vi "Connect.vi"(8 "error in":errorcluster, 11 "Luminos in":refnum<class "Luminos.lvclass">) -> (0 "error out":errorcluster, 3 "Luminos out":refnum<class "Luminos.lvclass">)   [LabVIEW 2018, in "Luminos.lvlib" / "Luminos.lvclass"]
uses:
  Luminos.lvclass
  PPLs/Axis/Axis.lvlibp/Axis.lvclass
  <instrlib>/ZaberTSeries/ZaberTSeries.lvlib
  C:/Projects/LabVIEW/PPLs/Axis/Axis.lvlibp/Axis.lvclass
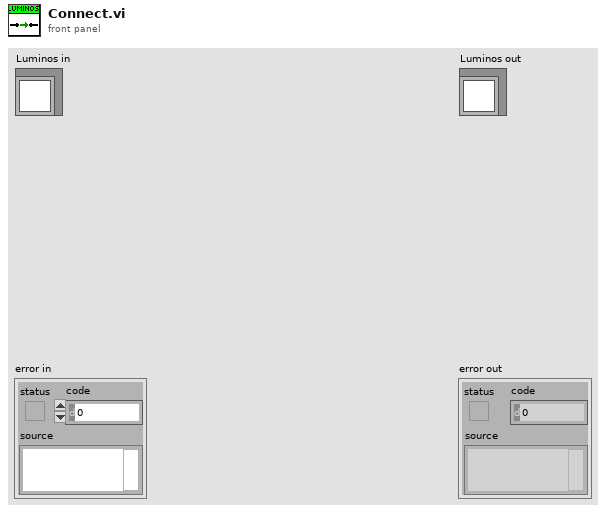
[diagram p1: front panel]
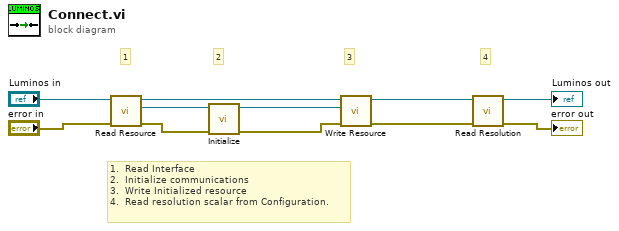
[diagram p0: block diagram]
diagram:
  # "1.  Read Interface\n2.  Initialize communications\n3.  Write Initialized resource \n4.  Read resolution scalar from Configuration."
  # "4"
  # "3"
  # "2"
  # "1"
  n1 = call "Read Resource.vi"("error in"="error in", "Axis in"="Luminos in") -> ("error out"=w1:errorcluster, "Resource"=w2:refnum<visa-resource-name>, "Axis out"=w10:refnum<class "Luminos.lvclass">)  [unwired: 7 in]
  n2 = call <instrlib>:"Initialize.vi"("error in (no error)"=w1, "VISA resource name"=w2) -> ("error out"=w8:errorcluster, "VISA resource name out"=w9:refnum<visa-resource-name>)  [unwired: 7 in, 1 out]
  n3 = call "Write Resource.vi"("error in"=w8, "Resource"=w9, "Axis in"=w10) -> ("error out"=w4:errorcluster, "Axis out"=w6:refnum<class "Luminos.lvclass">)  [unwired: 7 in]
  n4 = call "Read Resolution.vi"("error in"=w4, "Luminos in"=w6) -> ("error out"=→"error out":errorcluster, "Luminos out"=→"Luminos out":refnum<class "Luminos.lvclass">)  [unwired: 8 in]
